vi "Update Saving Status.vi"(8 "error in":errorcluster, 11 "File Actor in":refnum<class "File Actor.lvclass">) -> (0 "error out":errorcluster, 3 "File Actor out":refnum<class "File Actor.lvclass">)   [LabVIEW 2014, in "File Library.lvlib" / "File Actor.lvclass"]
doc: "This method of the File Actor object is used to tell the caller what the current file status is. This status generally will not differe from that directed by the caller, but in some cases, such as at configuration or if there is an error, the status may differ from that of the caller. \n\nThis VI is in community scope so it may be used by the Exe Write object to update when writing."
uses:
  File Actor.lvclass
  <vilib>/ActorFramework/Actor/Actor.lvclass/Actor.ctl
  File Actor.lvclass/File Actor.ctl
  Messages/Abstract/Saving File Message/Saving File Message.lvclass/Saving File Message.ctl
  <vilib>/ActorFramework/Message Enqueuer/Message Enqueuer.lvclass/Message Enqueuer.ctl
  Messages/Abstract/Saving File Message/Write Saving.vi
  <vilib>/ActorFramework/Message Priority Queue/Priority Enqueue.vi
  <vilib>/ActorFramework/Actor/Actor.lvclass
  <vilib>/ActorFramework/Message Enqueuer/Message Enqueuer.lvclass
  Messages/Abstract/Saving File Message/Saving File Message.lvclass
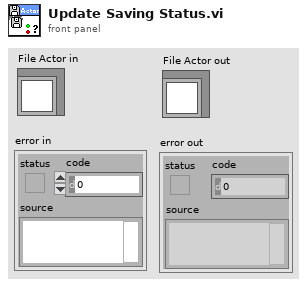
[diagram p1: front panel]
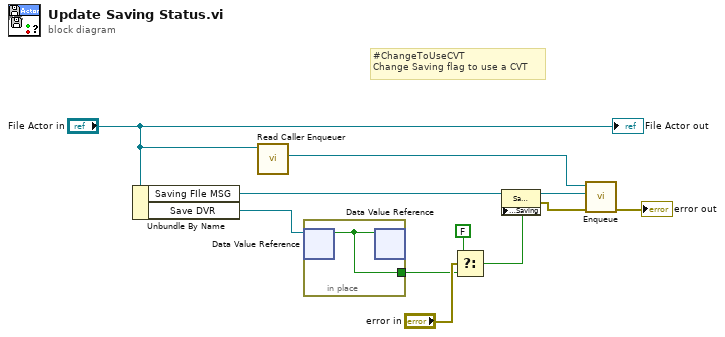
[diagram p0: block diagram]
diagram:
  # "#ChangeToUseCVT\nChange Saving flag to use a CVT"
  n1 = Unbundle By Name("File Actor in") -> ("Saving FIle MSG"=w2:refnum<class "Saving File Message.lvclass">, "Save DVR"=w11:refnum<data-value>)
  n2 = call <vilib>:"Read Caller Enqueuer.vi"("Actor"="File Actor in") -> ("Caller Enqueuer"=w9:refnum<class "Message Enqueuer.lvclass">)  [unwired: 10 in]
  n3 = in-place {
    in-place-border: [w12] -> w6
    n4 = in-place-dvr #1(w11) -> (w12:bool)  [unwired: 1 out]
    n5 = in-place-dvr #1(w12) -> ()  [unwired: 2 out]
  }
  n6 = Select(t=FALSE, s="error in", f=w6) -> (s? t:f=w4:bool)
  n7 = property class="Saving Main File MSG"(reference=w2, "Accessors:Saving"=w4) -> (reference out=w10:refnum<class "Saving File Message.lvclass">, error out=w1:errorcluster)  [unwired: 1 in]
  n8 = call <vilib>:"Enqueue.vi"("error in (no error)"=w1, "Message"=w10, "Message Enqueuer in"=w9) -> ("error out"=→"error out":errorcluster)  [unwired: 7 in, 1 out]
  "File Actor out" <- "File Actor in"
